vi "RRTPlan.vi"(10 "IA State":T5={"our_robots"=[], "enemy_robots"=[], "balls"=[], "geometry"={"line_width"=0, "field_length"=0, "field_width"=0, "boundary_width"=0, "referee_width"=0, "goal_width"=0, "goal_depth"=0, "goal_wall_width"=0, "center_circle_radius"=0, "defense_radius"=0, "defense_stretch"=0, "free_kick_from_defense_dist"=0, "penalty_spot_from_field_line_dist"=0, "penalty_line_from_spot_dist"=0}, "IA Judge"={"stage"="", "command"="", "our_goalie_id"=0.0, "enemy_goalie_id"=0.0, "command enum"=enum."Halt", "Time"=enum."Azul"}, "Received Timestamp"=timestamp(0 s since 1904-01-01), "Events"={"Touch"=FALSE, "Ball out"=FALSE, "id touch"=0.0, "Ball out of \nVision"=FALSE, "Ball inside \nGoalie area"=FALSE, "Robot not responding"=FALSE, "Robots responding status"=[1.0, 1.0, 1.0, 1.0, 1.0, 1.0], "Enemy Ball \nPossession"=FALSE, "Pass State"=FALSE, "id end of pass"=0.0, "Kick"=FALSE, "Id ini Possession"=0.0, "Ball Possesion"=FALSE, "Id Possesion"=0.0}}, 11 "Robot":T2={"id"=0, "function"=enum."Attacker", "x"=0.0, "y"=0.0, "orientation"=0.0, "v_tangent"=0.0, "v_normal"=0.0, "v_ang"=0.0, "kick_x"=0.0, "kick_z"=0.0, "dribble"=FALSE, "Timestamp"=timestamp(0 s since 1904-01-01), "dest_x"=0.0, "dest_y"=0.0, "dest_orientation"=0.0, "estimatives"={"est_v_tangent"=0.0, "est_v_normal"=0.0, "est_vx"=0.0, "est_vy"=0.0, "Pos Robot Est"=[]}, "dest_x_kick"=0.0, "dest_y_kick"=0.0, "Gap Coord"=[], "States"=enum."GoToTangent", "Path "=[]}) -> (2 "Robot Out":T2={"id"=0, "function"=enum."Attacker", "x"=0.0, "y"=0.0, "orientation"=0.0, "v_tangent"=0.0, "v_normal"=0.0, "v_ang"=0.0, "kick_x"=0.0, "kick_z"=0.0, "dribble"=FALSE, "Timestamp"=timestamp(0 s since 1904-01-01), "dest_x"=0.0, "dest_y"=0.0, "dest_orientation"=0.0, "estimatives"={"est_v_tangent"=0.0, "est_v_normal"=0.0, "est_vx"=0.0, "est_vy"=0.0, "Pos Robot Est"=[]}, "dest_x_kick"=0.0, "dest_y_kick"=0.0, "Gap Coord"=[], "States"=enum."GoToTangent", "Path "=[]})   [LabVIEW 2016]
uses:
  Core/AI Robot.ctl
  Intel/Functions Enum.ctl
  Intel/AttackerStates.ctl
  Core/AI Input.ctl
  Core/AI Ball.ctl
  Core/Field Size.ctl
  Core/AI Judge.ctl
  Intel/Command Enum.ctl
  Util/Events/Events.ctl
  <vilib>/Analysis/6fits.llb/1D B-Spline Fit.vi
  <vilib>/Analysis/NI_AALPro.lvlib
panel:
  out "Waveform Graph 3":dbl[](graph)
  out "Waveform Graph 2":dbl[](graph)
  out "Waveform Graph":dbl[](graph)
  out "size(s)":i32[](array[numeric])
  out "SplineY":i32
  out "SplineX":i32
  out "XY Graph":T1(graph)
  out "Best BSpline Fit X":dbl[](array[numeric])
  out "Best BSpline Fit Y":dbl[](array[numeric])
  out "x = y?":bool
  out "x = 0? 2":bool
  out "x = 0?":bool
  out "x > y?":bool
  out "SmoothPath":dbl[][](array[numeric])
  out "Time has Elapsed":bool
  out "Elapsed Time (s)":dbl
  in  "WayPointProb":dbl=0.6 format="%#_13g"
  in  "GoalProb":dbl=0.1 format="%#_13g"
  out "element":dbl
  in  "Step":dbl=80.0
  in  "threshold":dbl=20.0
  out "Goal":dbl[](array[numeric])
  out "Initial State":dbl[](array[numeric])
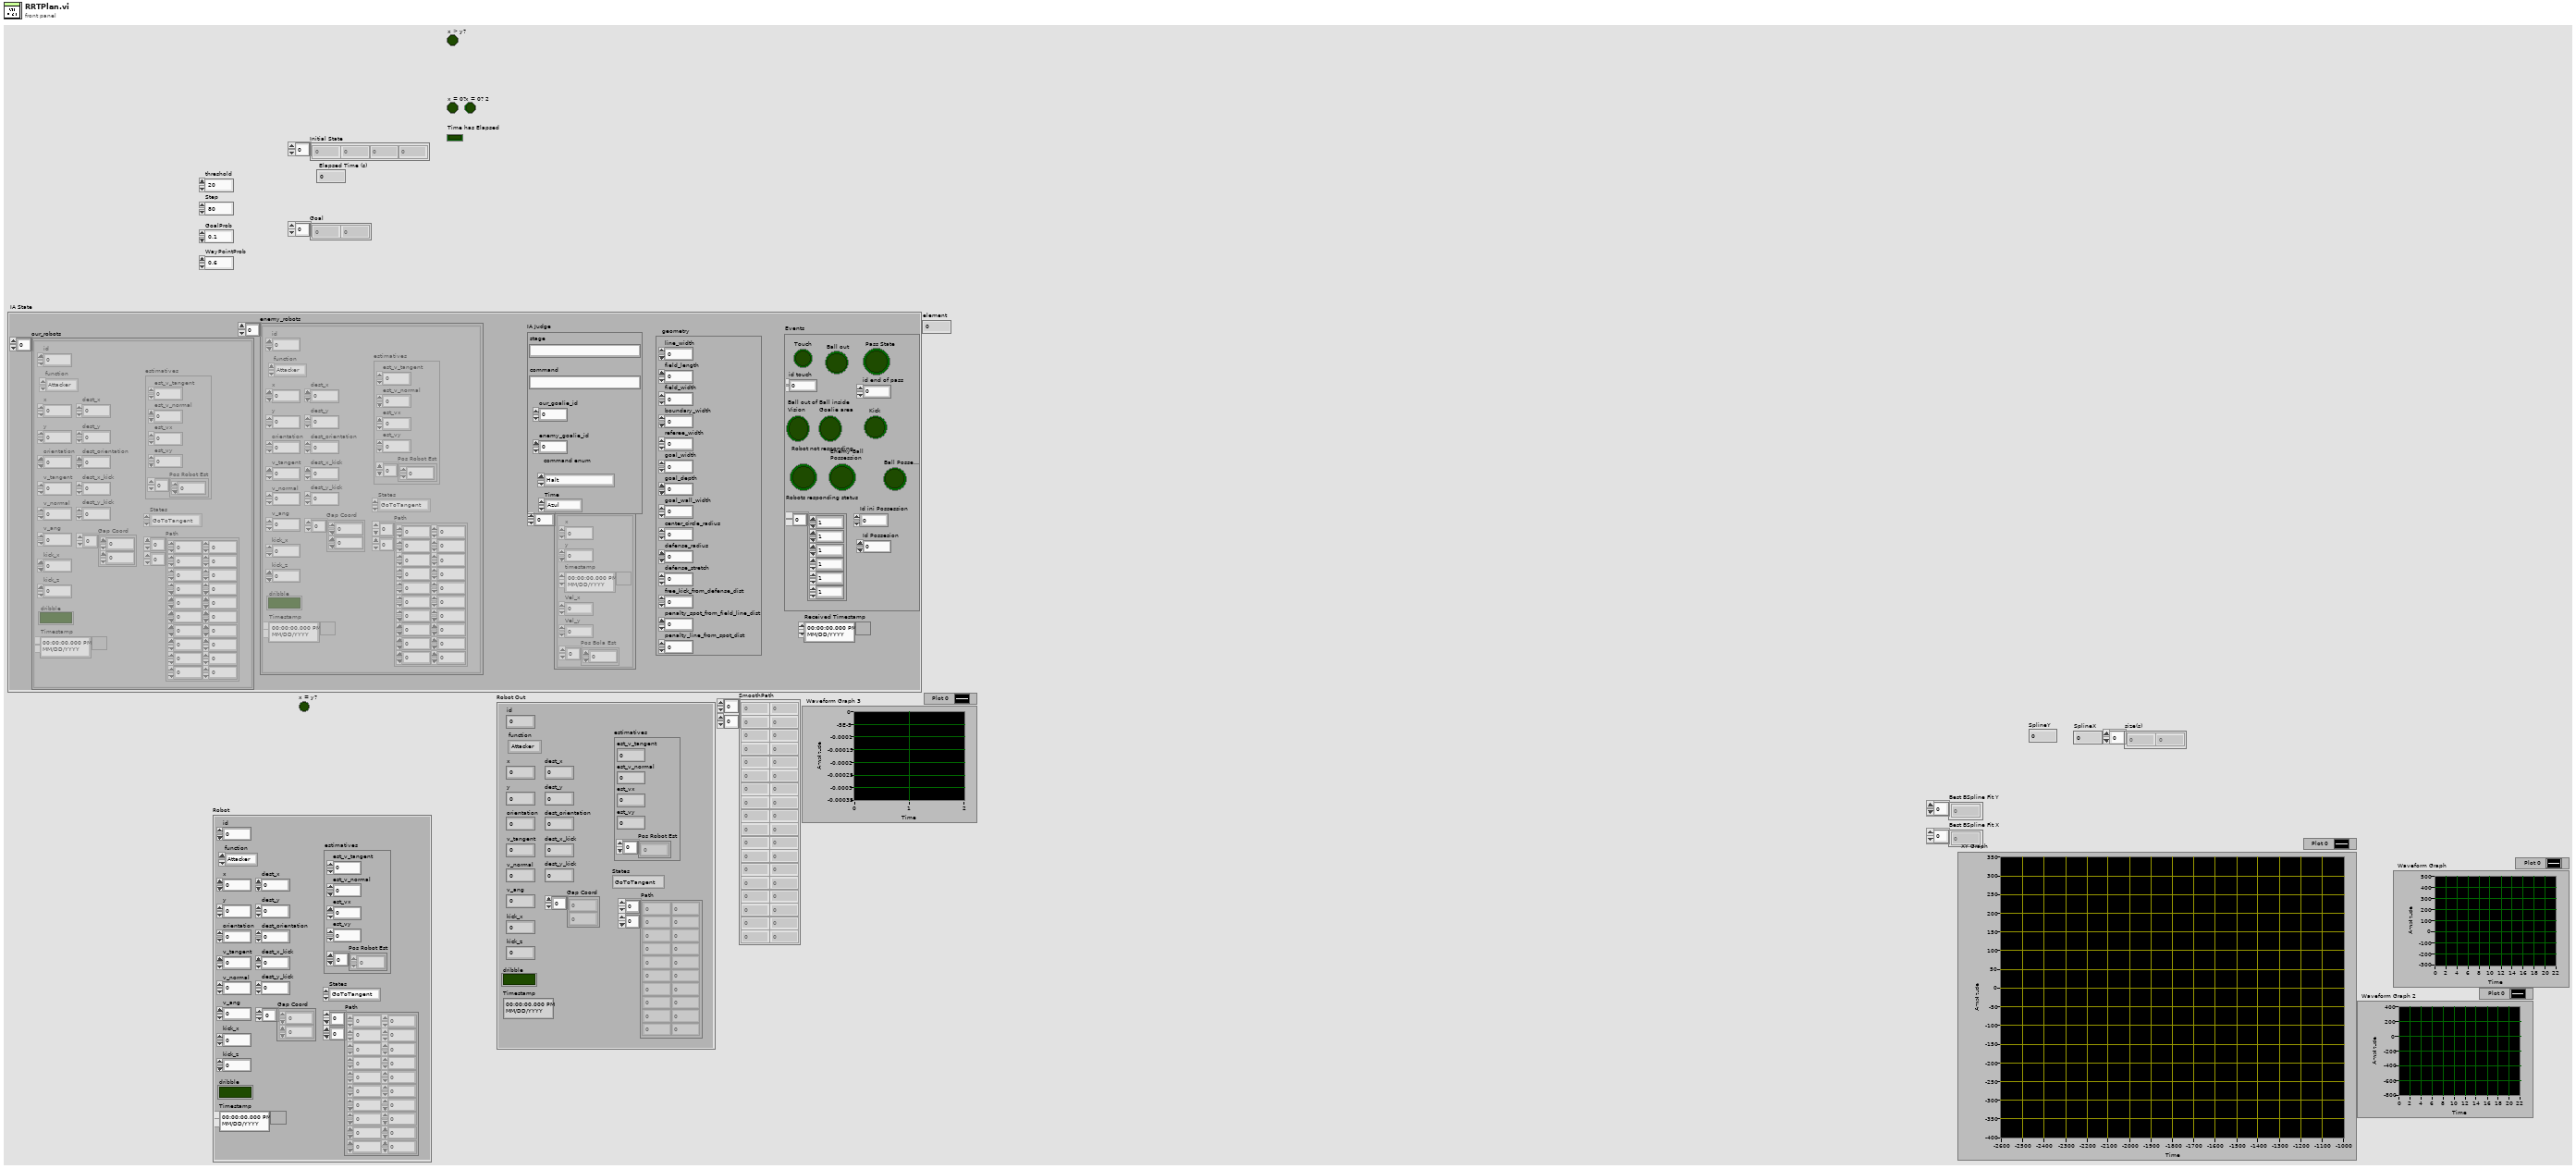
[diagram p1: front panel]
types:
  T1 = cluster{"SmoothPath":dbl[], "SmoothPath":dbl[]}[]
  T2 = typedef "AI Robot.ctl" = cluster{"id":u32, "function":T3, "x":dbl, "y":dbl, "orientation":dbl, "v_tangent":dbl, "v_normal":dbl, "v_ang":dbl, "kick_x":dbl, "kick_z":dbl, "dribble":bool, "Timestamp":timestamp, "dest_x":dbl, "dest_y":dbl, "dest_orientation":dbl, "estimatives":cluster{"est_v_tangent":dbl, "est_v_normal":dbl, "est_vx":dbl, "est_vy":dbl, "Pos Robot Est":dbl[]}, "dest_x_kick":dbl, "dest_y_kick":dbl, "Gap Coord":dbl[], "States":T4, "Path ":dbl[][]}
  T3 = typedef "Functions Enum.ctl" = enum16{"Attacker", "Goalie", "Defender", "Striker", "Goto 0", "Dummy", "Kicker", "ZigZag"}
  T4 = typedef "AttackerStates.ctl" = enum16{"Pass", "GoToTangent", "BallGetting", "GoToKick", ""}
  T5 = typedef "AI Input.ctl" = cluster{"our_robots":T2[], "enemy_robots":T2[], "balls":T6[], "geometry":T7, "IA Judge":T8, "Received Timestamp":timestamp, "Events":T10}
  T6 = typedef "AI Ball.ctl" = cluster{"x":dbl, "y":dbl, "timestamp":timestamp, "Vel_x":dbl, "Vel_y":dbl, "Pos Bola Est":dbl[]}
  T7 = typedef "Field Size.ctl" = cluster{"line_width":u32, "field_length":u32, "field_width":u32, "boundary_width":u32, "referee_width":u32, "goal_width":u32, "goal_depth":u32, "goal_wall_width":u32, "center_circle_radius":u32, "defense_radius":u32, "defense_stretch":u32, "free_kick_from_defense_dist":u32, "penalty_spot_from_field_line_dist":u32, "penalty_line_from_spot_dist":u32}
  T8 = typedef "AI Judge.ctl" = cluster{"stage":string, "command":string, "our_goalie_id":dbl, "enemy_goalie_id":dbl, "command enum":T9, "Time":enum16{"Azul", "Amarelo"}}
  T9 = typedef "Command Enum.ctl" = enum16{"Halt", "Stop", "Force Start", "PKA Normal Start", "Prepare Kickoff Ally", "PKE Normal Start", "Prepare Kickoff Enemy", "Prepare Penalty Ally", "PPA Normal Start", "Prepare Penalty Enemy", "PPE Normal Start", "Direct Free Enemy", "Direct Free Ally", "Indirect Free Enemy", "Indirect Free Ally", "Timeout Enemy", "Timeout Ally", "Goal Enemy", "Goal Ally", "Ball Placement Enemy", "Ball Placement Ally", "Normal Half Time", "Extra Time Break", "Extra Half Time", "None", "Post Game"}
  T10 = typedef "Events.ctl" = cluster{"Touch":bool, "Ball out":bool, "id touch":dbl, "Ball out of \nVision":bool, "Ball inside \nGoalie area":bool, "Robot not responding":bool, "Robots responding status":dbl[], "Enemy Ball \nPossession":bool, "Pass State":bool, "id end of pass":dbl, "Kick":bool, "Id ini Possession":dbl, "Ball Possesion":bool, "Id Possesion":dbl}
  T11 = cluster{"Best BSpline Fit X":dbl[], "Best BSpline Fit Y":dbl[]}
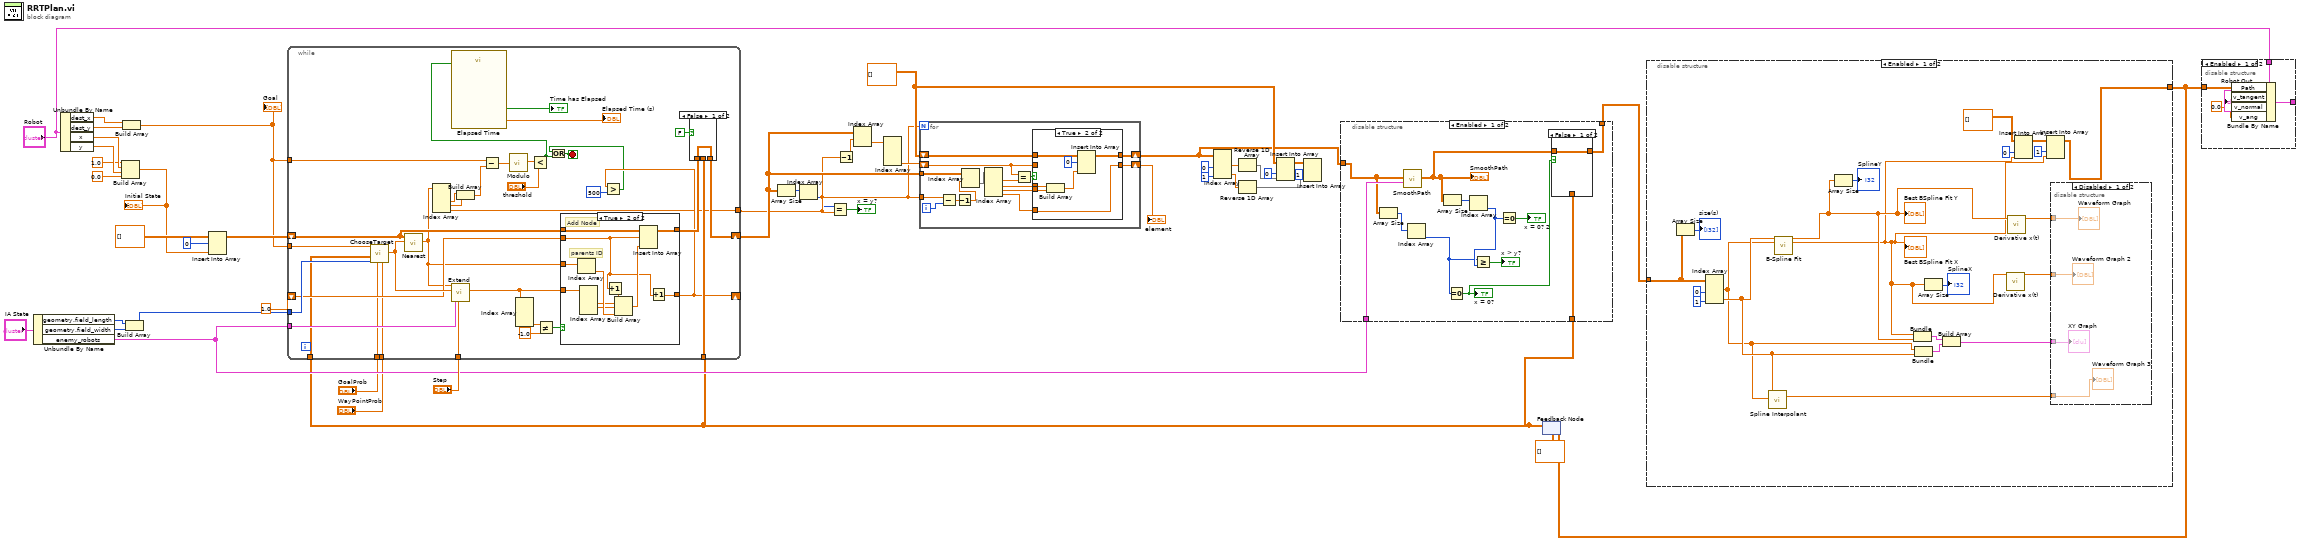
[diagram p0: block diagram]
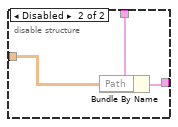
[diagram p4: hidden frame]
diagram:
  w15 = dbl[][] [] ("Path")
  n1 = Unbundle By Name("IA State") -> ("geometry.field_length"=w35:u32, "geometry.field_width"=w34:u32, "enemy_robots"=w24:T2[])
  n2 = Unbundle By Name("Robot") -> ("dest_x"=w41:dbl, "dest_y"=w40:dbl, "x"=w46:dbl, "y"=w45:dbl)
  n3 = Build Array(1.0 ("element"), w46, w45, 0.0 ("element")) -> (w39:dbl[])
  "Initial State" <- w39
  n4 = Build Array(w41, w40) -> (w37:dbl[])
  "Goal" <- w37
  n5 = Build Array(w35, w34) -> (w33:u32[])
  n6 = Insert Into Array(array=dbl[][] [] ("Pontos"), index (row)=0, new element=w39) -> (w38:dbl[][])  [unwired: 1 in]
  n7 = feedback #1(dbl[][] [] ("Path")) -> (w3:dbl[][])
  n8 = while {
    tunnel: w37 -> [w79]
    tunnel: w37 -> [w76]
    tunnel: w33 -> [w75]
    shift-right: [w57] -> w23
    shift-left: w38 -> [w56]
    tunnel: w24 -> [w73]
    tunnel: "Step" -> [w72]
    shift-right: [w53] -> _
    shift-left: 1.0 -> [w63]
    tunnel: w3 -> [w61]
    tunnel: w3 -> [w59]
    tunnel: "GoalProb" -> [w51]
    tunnel: "WayPointProb" -> [w50]
    tunnel: [w47] -> w5
    stop <- w67 stop-if-true
    n9 = call "ChooseTarget.vi"("WayPointProb"=w50, "GoalProb"=w51, "Field Geometry"=w75, "WayPointCache"=w61, "Goal"=w76) -> ("Target"=w74:dbl[])  [unwired: 6 in]
    n10 = call "Nearest.vi"("Target"=w74, "Pontos"=w56) -> ("Nearest"=w49:dbl[])  [unwired: 9 in]
    n11 = Index Array(array=w49) -> (element #2=w66:dbl, element #3=w65:dbl, element #4=w47:dbl)  [unwired: 4 in, 1 out]
    n12 = call "Extend.vi"("Step"=w72, "enemy_robots"=w73, "Target"=w74, "Nearest"=w49) -> ("New State"=w68:dbl[])  [unwired: 7 in]
    n13 = Build Array(w66, w65) -> (w64:dbl[])
    n14 = Subtract(x=w79, y=w64) -> (x-y=w80:dbl[])
    n15 = call "Modulo.vi"("2D vector"=w80) -> ("Modulo"=w78:dbl)  [unwired: 10 in]
    n16 = Index Array(array=w68) -> (element #4=w71:dbl)  [unwired: 4 in, 3 out]
    n17 = Less?(x=w78, y="threshold") -> (x < y?=w60:bool)
    n18 = call "Elapsed Time"("Reset"=w60) -> ("Elapsed Time (s)"=→"Elapsed Time (s)":dbl, "Time has Elapsed"=→"Time has Elapsed":bool)  [unwired: 11 in, 6 out]
    n19 = Not Equal?(x=w71, y=-1.0) -> (x != y?=w69:bool)
    n20 = case shown="True" w69 {
      tunnel: w56 -> [w84 w95]
      tunnel: [w84 w90] -> w58
      tunnel: w68 -> [_ w94]
      tunnel: w63 -> [w83 w86]
      tunnel: w49 -> [_ w92]
      tunnel: [w83 w87] -> w53
      frame False {
      }
      frame True {
        # "Add Node"
        # "parents ID"
        n21 = Index Array(array=w92) -> (element=w91:dbl)  [unwired: 1 in]
        n22 = Index Array(array=w94) -> (element #2=w89:dbl, element #3=w88:dbl)  [unwired: 4 in, 2 out]
        n23 = Increment(x=w86) -> (x+1=w85:dbl)
        n24 = Build Array(w85, w89, w88, w91) -> (w93:dbl[])
        n25 = Insert Into Array(array=w95, index (row)=w86, new element=w93) -> (w90:dbl[][])  [unwired: 1 in]
        n26 = Increment(x=w86) -> (x+1=w87:dbl)
      }
    }
    n27 = Greater?(x=w53, y=500) -> (0:w48:bool)
    n28 = Or(x=w48, y=w60) -> (x .or. y?=w67:bool)
    n29 = case shown="False" FALSE {
      tunnel: w59 -> [_ w82]
      tunnel: [w81 w82] -> w57
      tunnel: w58 -> [w81 _]
      frame False {
      }
      frame True {
      }
    }
  }
  n30 = Array Size(array=w23) -> (size(s)=w31:i32[])
  n31 = Index Array(array=w31) -> (element=w4:i32)  [unwired: 1 in]
  n32 = Equal?(x=w4, y=w5) -> (x = y?=→"x = y?":bool)
  n33 = Decrement(x=w5) -> (x-1=w20:dbl)
  n34 = Index Array(array=w23, index (row)=w20) -> (element=w22:dbl[])  [unwired: 1 in]
  n35 = Index Array(array=w22) -> (element #4=w21:dbl)  [unwired: 4 in, 3 out]
  n36 = for {
    N: w5 -> [_]
    shift-right: [w106] -> w7
    shift-left: w15 -> [w107]
    tunnel: w5 -> [w105]
    tunnel: w23 -> [w103]
    shift-right: [w100] -> w30
    shift-left: w21 -> [w98]
    i -> [w104]
    n37 = Subtract(x=w105, y=w104) -> (x-y=w97:dbl)
    n38 = Decrement(x=w97) -> (x-1=w96:dbl)
    n39 = Index Array(array=w103, index (row)=w96) -> (element=w102:dbl[])  [unwired: 1 in]
    n40 = Index Array(array=w102) -> (element #1=w101:dbl, element #2=w109:dbl, element #3=w108:dbl, element #4=w99:dbl)  [unwired: 4 in]
    n41 = Equal?(x=w98, y=w101) -> (x = y?=w110:bool)
    n42 = case shown="True" w110 {
      tunnel: w109 -> [_ w119]
      tunnel: w108 -> [_ w118]
      tunnel: w107 -> [w112 w117]
      tunnel: [w112 w115] -> w106
      tunnel: [w111 w114] -> w100
      tunnel: w99 -> [_ w114]
      tunnel: w98 -> [w111 _]
      frame False {
      }
      frame True {
        n43 = Build Array(w119, w118) -> (w116:dbl[])
        n44 = Insert Into Array(array=w117, index (row)=0, new element=w116) -> (w115:dbl[][])  [unwired: 1 in]
      }
    }
  }
  "element" <- w30
  n45 = Index Array(array=w7, index (col) #1=0 ("disabled index (col)"), index (col) #2=1 ("index (col)")) -> (element #1=w17:dbl[], element #2=w16:dbl[])  [unwired: 2 in]
  n46 = Reverse 1D Array(array=w16) -> (reversed array=w10:dbl[])
  n47 = Reverse 1D Array(array=w17) -> (reversed array=w14:dbl[])
  n48 = Insert Into Array(array=w15, index (col)=0 ("disabled index (col)"), new element=w14) -> (w12:dbl[][])  [unwired: 1 in]
  n49 = Insert Into Array(array=w12, index (col)=1 ("disabled index (col)"), new element=w10) -> ()  [unwired: 1 in, 1 out]
  n50 = disable-structure shown="Enabled" {
    disable-tunnel: w24 -> [w131 _]
    disable-tunnel: w7 -> [w124 w134]
    disable-tunnel: [w120 w134] -> w2
    disable-tunnel: w3 -> [w122 _]
    frame Enabled {
      n51 = Array Size(array=w124) -> (size(s)=w129:i32[])
      n52 = call "SmoothPath.vi"("enemy_robots"=w131, "Path"=w124) -> ("SmoothPath"=w121:dbl[][])  [unwired: 9 in]
      "SmoothPath" <- w121
      n53 = Index Array(array=w129) -> (element=w126:i32)  [unwired: 1 in]
      n54 = Array Size(array=w121) -> (size(s)=w130:i32[])
      n55 = Equal To 0?(x=w126) -> (x = 0?=w123:bool)
      "x = 0?" <- w123
      n56 = Index Array(array=w130) -> (element=w127:i32)  [unwired: 1 in]
      n57 = Greater Or Equal?(x=w126, y=w127) -> (x >= y?=→"x > y?":bool)
      n58 = Equal To 0?(x=w127) -> (x = 0?=→"x = 0? 2":bool)
      n59 = case shown="False" w123 {
        tunnel: w122 -> [_ w133]
        tunnel: [w132 w133] -> w120
        tunnel: w121 -> [w132 _]
        frame False {
        }
        frame True {
        }
      }
    }
    frame Disabled {
    }
  }
  n60 = disable-structure shown="Enabled" {
    disable-tunnel: w2 -> [w142 w160]
    disable-tunnel: [w136 w160] -> w1
    frame Enabled {
      n61 = Array Size(array=w142) -> (size(s)=→"size(s)":i32[])
      n62 = Index Array(array=w142, index (col) #1=0 ("disabled index (col)"), index (col) #2=1 ("index (col)")) -> (element #1=w146:dbl[], element #2=w147:dbl[])  [unwired: 2 in]
      n63 = call <vilib>:"Spline Interpolant.vi"("X"=w146, "Y"=w147) -> ("Interpolant"=w135:dbl[])  [unwired: 2 in, 1 out]
      n64 = call-poly <vilib>:"B-Spline Fit.vi"("Y"=w147, "X"=w146) -> ("Best BSpline Fit Y"=w145:dbl[], "Best BSpline Fit X"=w137:dbl[])  [unwired: 10 in, 2 out]
      "Best BSpline Fit Y" <- w145
      "Best BSpline Fit X" <- w137
      n65 = Array Size(array=w145) -> (size(s)=→"SplineY":i32)
      n66 = Bundle("Best BSpline Fit X"=w137, "Best BSpline Fit Y"=w145) -> (w153:T11)  [unwired: 1 in]
      n67 = Bundle("Path"=w146, "Path"=w147) -> (w152:cluster{"Path":dbl[], "Path":dbl[]})  [unwired: 1 in]
      n68 = Array Size(array=w137) -> (size(s)=→"SplineX":i32)
      n69 = Build Array(w153, w152) -> (w151:cluster{"Path":dbl[], "Path":dbl[]}[])
      n70 = call <vilib>:"Derivative x(t).vi"("X"=w137) -> ("dX/dt"=w144:dbl[])  [unwired: 9 in, 1 out]
      n71 = call <vilib>:"Derivative x(t).vi"("X"=w145) -> ("dX/dt"=w143:dbl[])  [unwired: 9 in, 1 out]
      n72 = Insert Into Array(array=dbl[][] [] ("Path"), index (col)=0 ("disabled index (col)"), new element=w137) -> (w139:dbl[][])  [unwired: 1 in]
      n73 = Insert Into Array(array=w139, index (col)=1 ("disabled index (col)"), new element=w137) -> (w136:dbl[][])  [unwired: 1 in]
      n74 = disable-structure shown="Disabled" {
        disable-tunnel: w151 -> [w159 _]
        disable-tunnel: w144 -> [w158 _]
        disable-tunnel: w143 -> [w157 _]
        disable-tunnel: w135 -> [w156 _]
        frame Disabled {
          "XY Graph" <- w159
          "Waveform Graph" <- w157
          "Waveform Graph 2" <- w158
          "Waveform Graph 3" <- w156
        }
        frame Enabled {
        }
      }
    }
    frame Disabled {
    }
  }
  n75 = feedback-in #1(w1) -> ()
  n76 = disable-structure shown="Enabled" {
    disable-tunnel: "Robot" -> [w164 w166]
    disable-tunnel: [w163 w167] -> w28
    disable-tunnel: w1 -> [w162 w165]
    frame Enabled {
      w161 = 0.0 ("v_normal")
      n77 = Bundle By Name(cluster=w164, "Path"=w162, "v_tangent"=w161, "v_normal"=w161, "v_ang"=w161) -> (w163:T2)
    }
    frame Disabled {
      n78 = Bundle By Name(cluster=w166, "Path"=w165) -> (w167:T2)
    }
  }
  "Robot Out" <- w28
